vi "2signal.vi"(8 "데이터":string, 9 "Dat.Num":string, 10 "커맨드":string, 11 "국번":string) -> (3 "String":string)   [LabVIEW 2013]
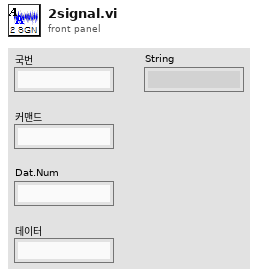
[diagram p1: front panel]
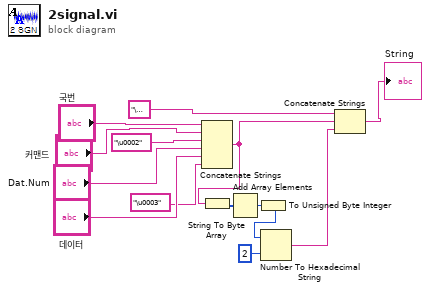
[diagram p0: block diagram]
diagram:
  n1 = Concatenate Strings("국번", "커맨드", "\u0002", "Dat.Num", "데이터", "\u0003") -> (w7:string)
  n2 = String To Byte Array(string=w7) -> (unsigned byte array=w8:u8[])
  n3 = Add Array Elements(numeric array=w8) -> (sum=w9:u8)
  n4 = To Unsigned Byte Integer(number=w9) -> (unsigned 8bit integer=w2:u8)
  n5 = Number To Hexadecimal String(1:i16 2 ("폭(-)"), 2:w2) -> (0:w6:string)
  n6 = Concatenate Strings("\u0001", w7, w6) -> (→"String":string)
